vi "Init Message Transport Event.vi"(8 "error in (no error)":errorcluster, 11 "Event":refnum<class "Message Interface.lvclass">) -> (0 "error out":errorcluster, 3 "Message Transport Event out":refnum<class "Message Transport Event.lvclass">)   [LabVIEW 2016, in "Stream Mediator.lvlib" / "Message Transport Event.lvclass"]
doc: "--\nCopyright © 2017 Composed SystemsI All rights reserved.\n\nAuthor: Jon McBee <jon.mcbee@composed.io>\n\nThis library is provided \"AS IS\" ,WITHOUT WARRANTIES OR\nCONDITIONS OF ANY KIND, either express or implied.\n\nComposed Systems -- composed.io\n\nStream 0.0.1.1\nJon McBee - Composed Systems\nCopyright (c) 2017, Composed Systems"
uses:
  <userlib>/Composed Systems/Stream/Mediator/Classes/Message Transport Event/Message Transport Event.lvclass
  <userlib>/Composed Systems/Stream/Mediator/Classes/Message Interface/Message Interface.lvclass
  <userlib>/Composed Systems/Stream/Mediator/Classes/Message Transport Event/Message Transport Event.lvclass/Message Transport Event.ctl
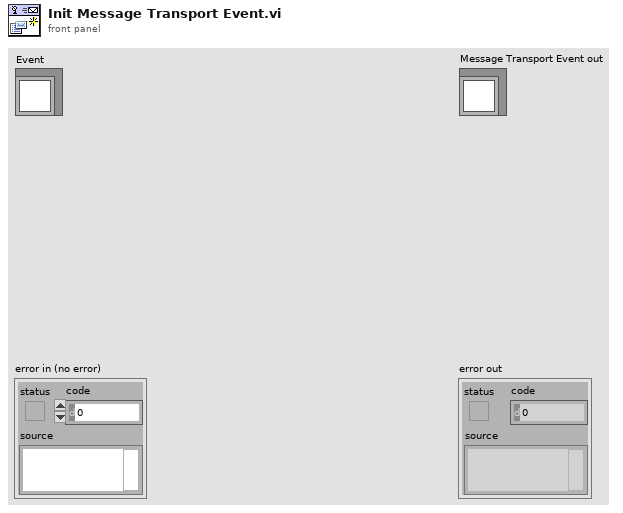
[diagram p1: front panel]
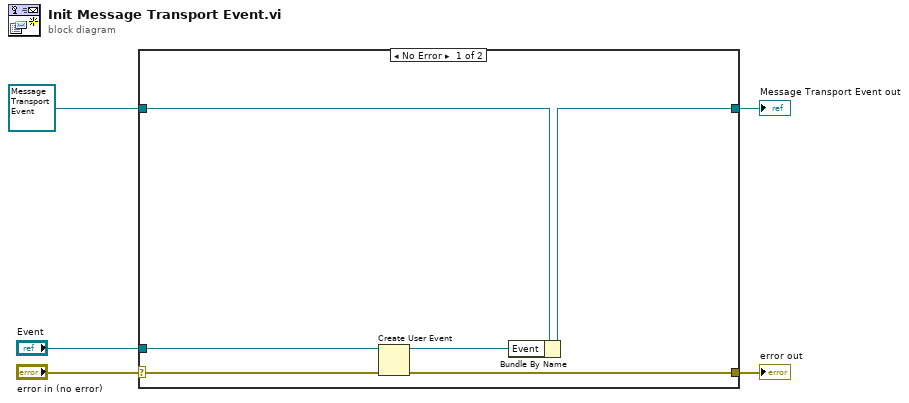
[diagram p0: block diagram]
diagram:
  n1 = case shown="No Error" "error in (no error)" {
    selector: "error in (no error)" -> [w11 w13]
    tunnel: [w10 w13] -> w4
    tunnel: [w8 w12] -> w2
    tunnel: refnum<class "Message Transport Event.lvclass"> refnum ("Message Transport Event in") -> [w9 w12]
    tunnel: "Event" -> [w7 _]
    frame No Error {
      n2 = Create User Event(user event datatype=w7, error in=w11) -> (user event=w6:refnum<user-event>, error out=w10:errorcluster)
      n3 = Bundle By Name(cluster=w9, "Event"=w6) -> (w8:refnum<class "Message Transport Event.lvclass">)
    }
    frame Error {
    }
  }
  "error out" <- w4
  "Message Transport Event out" <- w2
